vi "zc_tk.vi"(0 "id":string, 1 "LabVIEW Web Service Request":refnum<class "Web Request.lvclass"> caption="LabVIEW Web服务请求", 2 "sp_shuoming":string, 3 "lc_num":string, 5 "action":string, 7 "zc_luodi_num":string, 9 "shuoming":string, 11 "jsren":string, 12 "didian":string, 14 "sp_yijian":string, 15 "key":string) -> (10 "error":errorcluster)   [LabVIEW 2017]
uses:
  <vilib>/wsapi/Web Request.lvclass
panel:
  in  "error 3":errorcluster={"status"=TRUE, "code"=255, "source"="当前资产不是“领用”状态！"} caption="error"
  out "postdata":string caption="post数据"
  out "error out":errorcluster caption="错误输出"
  # "Web服务请求输入接线端用于调用“Web服务”选板的VI。除非不需要访问该选板，否则不要在连线板上删除这个输入接线端。"
  # "添加至连线板的每一个其他输入控件，在URL中对应于一个输入。如需在接线端模式输出（默认设置）下包含显示控件，则该显示控件必须与连线板相连。"
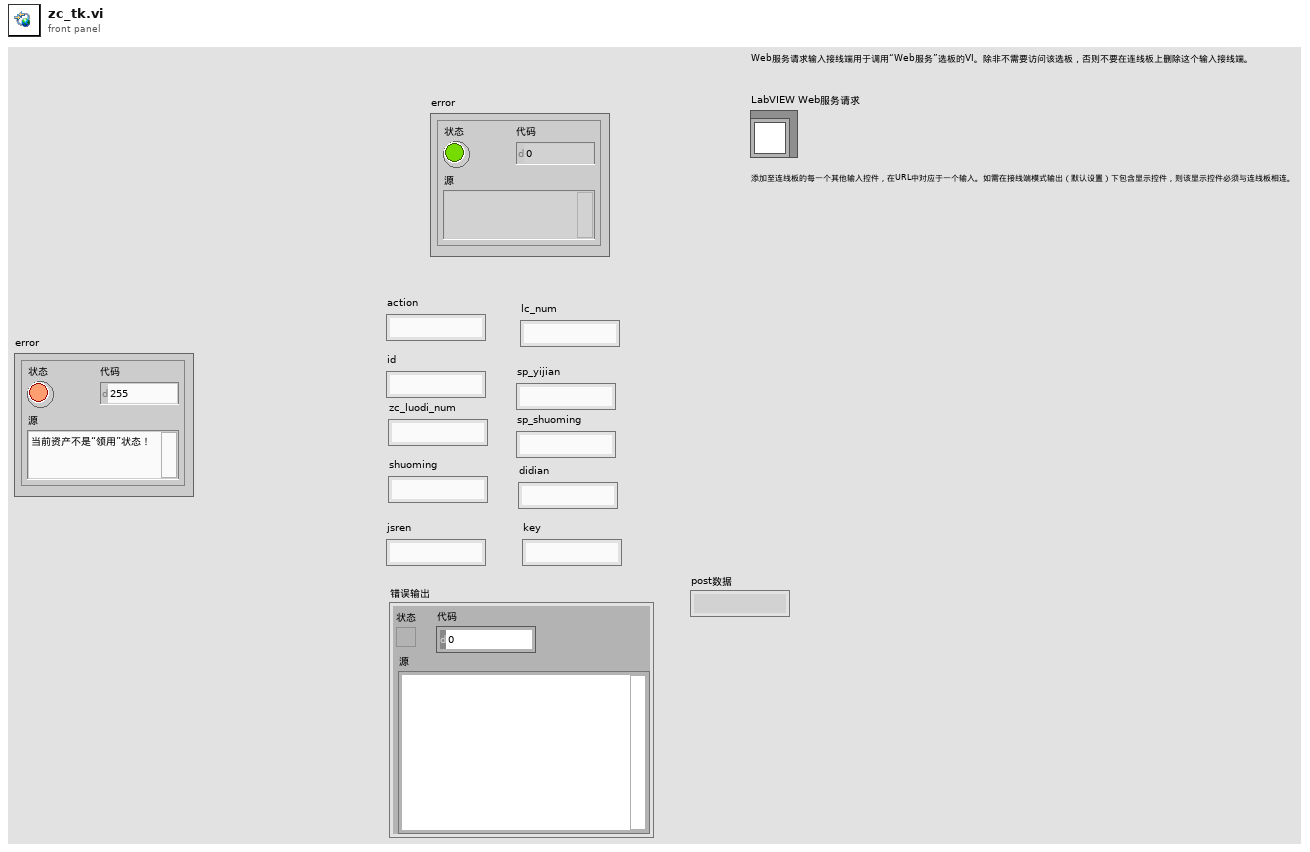
[diagram p1: front panel]
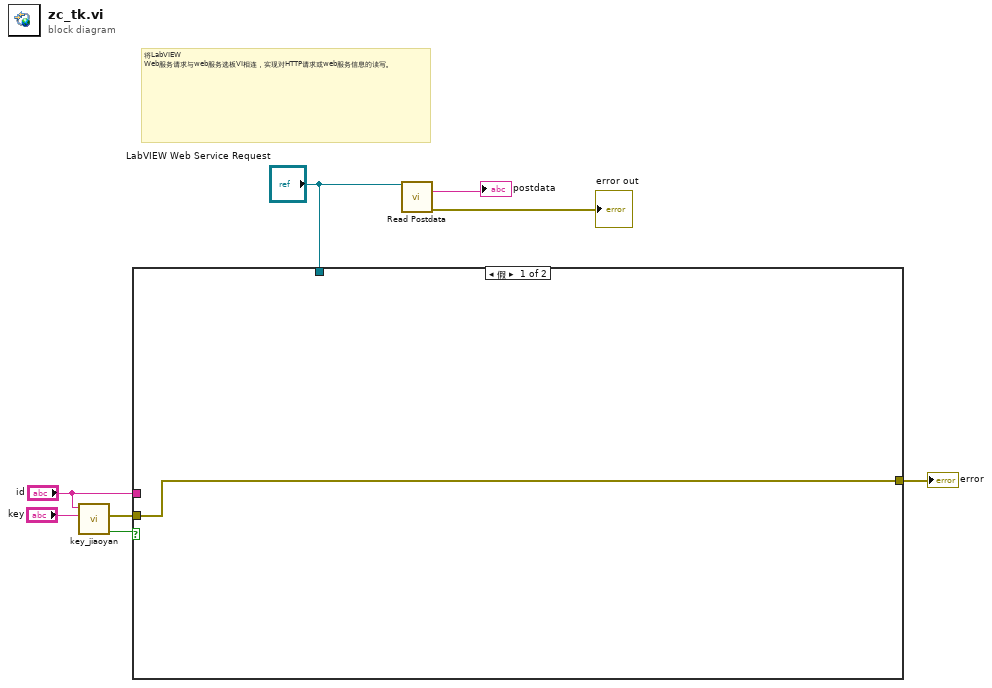
[diagram p0: block diagram]
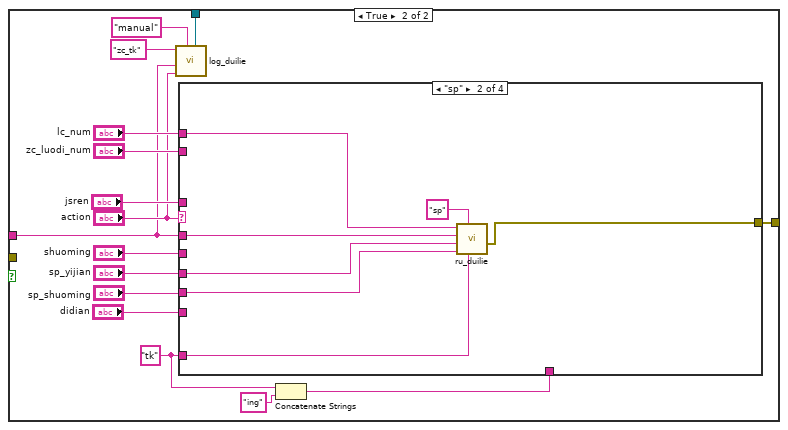
[diagram p2: hidden frame]
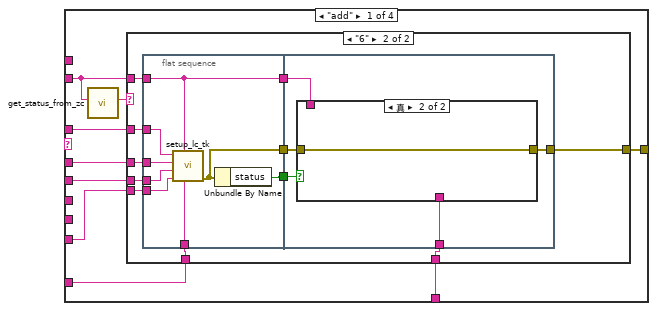
[diagram p3: hidden frame]
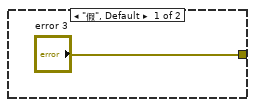
[diagram p4: hidden frame]
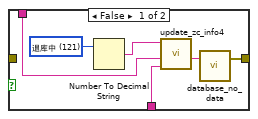
[diagram p5: hidden frame]
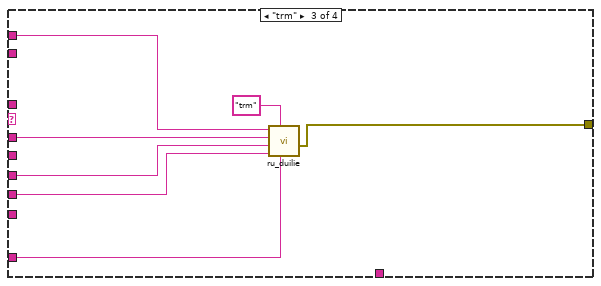
[diagram p6: hidden frame]
diagram:
  # "将LabVIEW Web服务请求与web服务选板VI相连，实现对HTTP请求或web服务信息的读写。"
  n1 = call "key_jiaoyan.vi"("key_client"="key", "gonghao"="id") -> ("jy"=w2:bool, "error"=w1:errorcluster)  [unwired: 8 in]
  n2 = case shown="假" w2 {
    tunnel: [w9 w20] -> w7
    tunnel: "LabVIEW Web Service Request" -> [_ w14]
    tunnel: "id" -> [_ w10]
    tunnel: w1 -> [w9 _]
    frame False {
    }
    frame True {
      w18 = "tk" ("yw")
      n3 = call "log_duilie.vi"("LabVIEW Web Service Request"=w14, "type"="manual", "action"="action", "user"=w10, "yw"="zc_tk") -> ()  [unwired: 7 in]
      n4 = Concatenate Strings(w18, "ing" ("字符串")) -> (w17:string)
      n5 = case shown="\"sp\"" "action" {
        tunnel: w10 -> [w34 w71 w78 _]
        tunnel: "zc_luodi_num" -> [w27 _ _ _]
        tunnel: "lc_num" -> [_ w72 w79 _]
        tunnel: "sp_yijian" -> [_ w70 w77 _]
        tunnel: "sp_shuoming" -> [_ w69 w76 _]
        tunnel: w18 -> [w32 w68 w75 _]
        tunnel: "shuoming" -> [w33 _ _ _]
        tunnel: [w31 w67 w74 _] -> w20
        tunnel: w17 -> [w30 _ _ _]
        tunnel: "didian" -> [w29 _ _ _]
        tunnel: "jsren" -> [w28 _ _ _]
        frame "add" {
          n6 = call "get_status_from_zc.vi"("zc_luodi_num"=w27) -> ("status"=w26:string)  [unwired: 9 in, 1 out]
          n7 = case shown="\"6\"" w26 {
            tunnel: w27 -> [_ w45]
            tunnel: w34 -> [_ w44]
            tunnel: w33 -> [_ w43]
            tunnel: w32 -> [_ w42]
            tunnel: ["error 3" w41] -> w31
            tunnel: w30 -> [_ w40]
            tunnel: w29 -> [_ w39]
            tunnel: w28 -> [_ w38]
            frame "假", Default {
            }
            frame "6" {
              n8 = flat-sequence {
                tunnel: [w50] -> w46
                tunnel: w45 -> [w50]
                tunnel: w44 -> [w54]
                tunnel: w43 -> [w53]
                tunnel: w42 -> [w52]
                tunnel: w39 -> [w51]
                tunnel: w38 -> [w49]
                tunnel: [w48] -> w37
                tunnel: [w47] -> w36
                tunnel: w46 -> [w58]
                tunnel: [w59] -> w41
                tunnel: w40 -> [w57]
                tunnel: w37 -> [w56]
                tunnel: w36 -> [w55]
                frame #0 {
                  n9 = call "setup_lc_tk.vi"("yw"=w52, "zc_luodi_num"=w50, "didian"=w51, "shuoming"=w53, "id"=w54, "jsren"=w49) -> ("error"=w47:errorcluster)  [unwired: 5 in]
                  n10 = Unbundle By Name(w47) -> ("status"=w48:bool)
                }
                frame #1 {
                  n11 = case shown="真" w56 {
                    tunnel: [w63 w66] -> w59
                    tunnel: w58 -> [w61 _]
                    tunnel: w57 -> [w60 _]
                    tunnel: w55 -> [_ w66]
                    frame False {
                      w62 = u8 121 items=["待验收"=1, "无需验收"=2, "验收不合格"=3, "待入库"=4, "入库"=5, "领用"=6, "借用"=7, "托管"=8, "接管"=9, "退出"=10, "出库在用"=11, "盘亏"=12, "出售"=13, "报废"=14, "领用中"=120, "退库中"=121, "借用中"=122, "归还中"=123, "转移中"=124, "调拨中"=125, "借调中"=126, "托管中"=127, "终止托管中"=128, "退出中"=129, "处置中"=130] ("状态选择器")
                      n12 = Number To Decimal String(number=w62) -> (decimal integer string=w64:string)  [unwired: 1 in]
                      n13 = call "update_zc_info4.vi"("ywxinxi"=w60, "number"=w61, "status"=w64) -> ("data_str"=w65:string)  [unwired: 8 in]
                      n14 = call "database_no_data.vi"("input"=w65) -> ("error"=w63:errorcluster)  [unwired: 2 in]
                    }
                    frame True {
                    }
                  }
                }
              }
            }
          }
        }
        frame "sp" {
          n15 = call "ru_duilie.vi"("yw"=w68, "name"="sp" ("元素"), "sp_shuoming"=w69, "sp_yijian"=w70, "id"=w71, "lc_num"=w72) -> ("error"=w67:errorcluster)  [unwired: 5 in]
        }
        frame "trm" {
          n16 = call "ru_duilie.vi"("yw"=w75, "name"="trm" ("元素"), "sp_shuoming"=w76, "sp_yijian"=w77, "id"=w78, "lc_num"=w79) -> ("error"=w74:errorcluster)  [unwired: 5 in]
        }
        frame Default {
        }
      }
    }
  }
  "error" <- w7
  n17 = call <vilib>:"Read Postdata.vi"("LabVIEW Web Service Request"="LabVIEW Web Service Request") -> ("postdata"=→"postdata":string, "error out"=→"error out":errorcluster)  [unwired: 12 in, 1 out]
